vi "L07.vi"() -> ()   [LabVIEW 2012]
panel:
  out "size(s)":i32
  out "Array 2":i32[](array[numeric])
  out "Array":bool[](array[boolean])
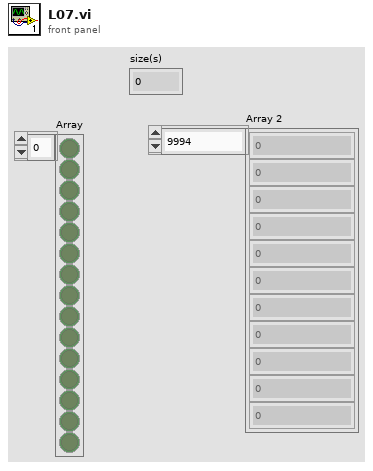
[diagram p1: front panel]
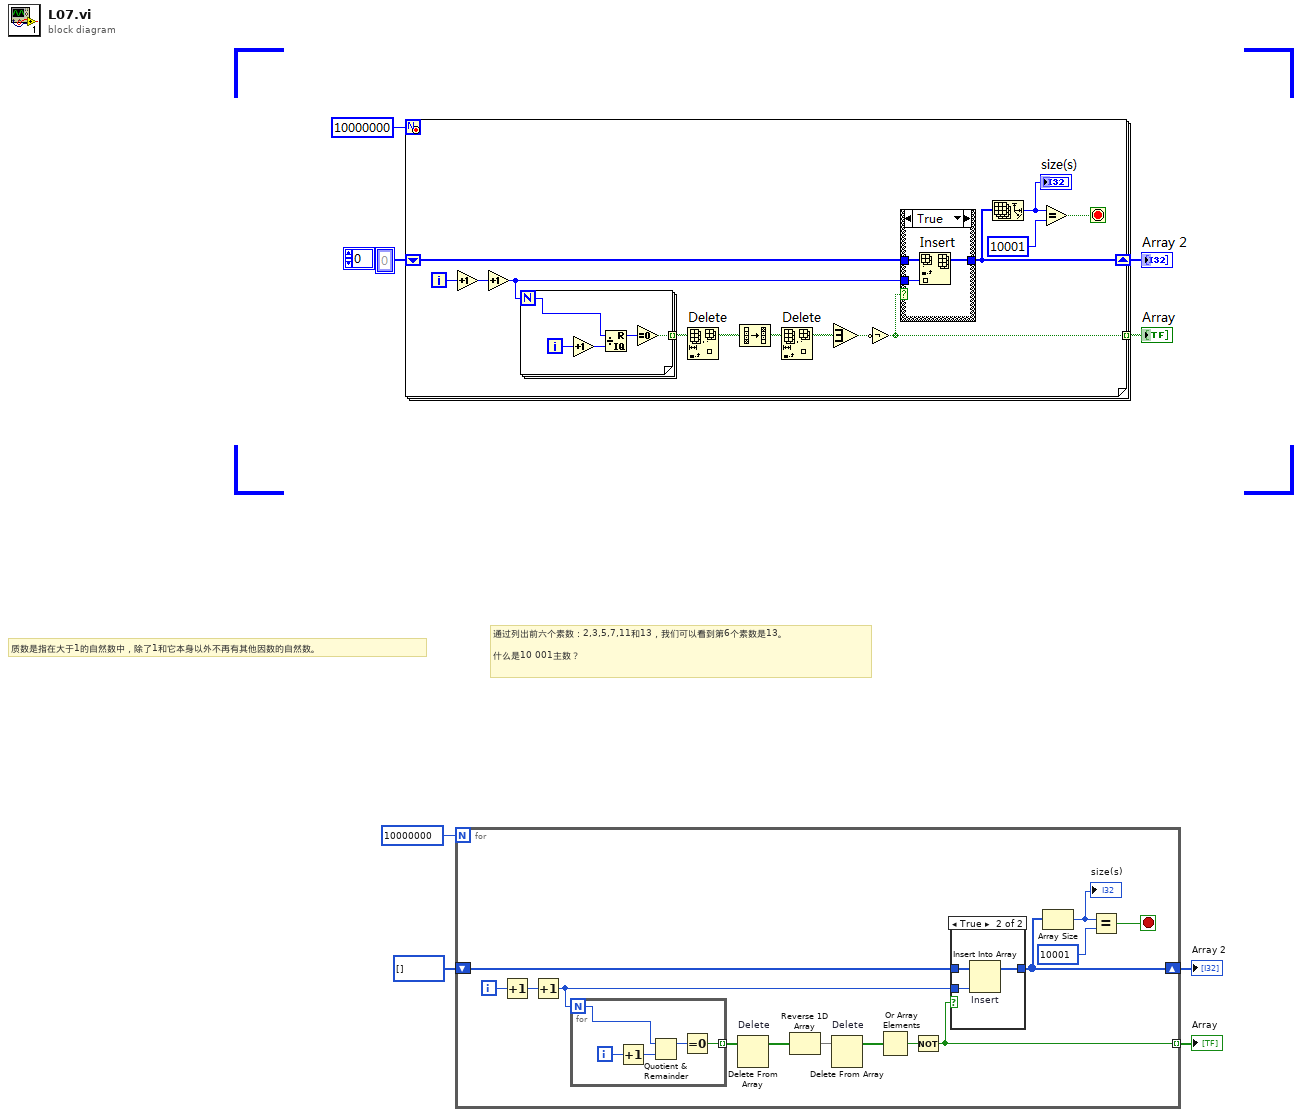
[diagram p0: block diagram]
diagram:
  # "通过列出前六个素数：2,3,5,7,11和13，我们可以看到第6个素数是13。\n\n什么是10 001主数？"
  # "质数是指在大于1的自然数中，除了1和它本身以外不再有其他因数的自然数。"
  n1 = for {
    N: 10000000 -> [_]
    tunnel: [w8] -> w3 mode=indexing
    shift-right: [w5] -> w1
    shift-left: i32[] [] -> [w7]
    i -> [w13]
    stop <- w9 stop-if-true
    n2 = Increment(x=w13) -> (x+1=w12:i32)
    n3 = Increment(x=w12) -> (x+1=w6:i32)
    n4 = for {
      N: w6 -> [w25]
      tunnel: [w26] -> w18 mode=indexing
      i -> [w24]
      n5 = Increment(x=w24) -> (x+1=w23:i32)
      n6 = Quotient & Remainder(x=w25, y=w23) -> (x-y*floor(x/y)=w27:i32)  [unwired: 1 out]
      n7 = Equal To 0?(x=w27) -> (x = 0?=w26:bool)
    }
    n8 = Delete From Array "Delete"(array=w18) -> (array with subset deleted=w17:bool[])  [unwired: 2 in, 1 out]
    n9 = Reverse 1D Array(array=w17) -> (reversed array=w16:bool[])
    n10 = Delete From Array "Delete"(array=w16) -> (array with subset deleted=w15:bool[])  [unwired: 2 in, 1 out]
    n11 = Or Array Elements(Boolean array=w15) -> (logical OR=w14:bool)
    n12 = Not(x=w14) -> (.not. x?=w8:bool)
    n13 = case shown="True" w8 {
      tunnel: w7 -> [w19 w22]
      tunnel: [w19 w21] -> w5
      tunnel: w6 -> [_ w20]
      frame False {
      }
      frame True {
        n14 = Insert Into Array "Insert"(array=w22, new element=w20) -> (w21:i32[])  [unwired: 1 in]
      }
    }
    n15 = Array Size(array=w5) -> (size(s)=w11:i32)
    "size(s)" <- w11
    n16 = Equal?(x=w11, y=10001) -> (x = y?=w9:bool)
  }
  "Array" <- w3
  "Array 2" <- w1
